vi "Stim Train Log String.vi"(1 "Single Channel Params":T1 {"Train Length" min=20 max=500 step=5}) -> (0 "Stim Train Log String":string)   [LabVIEW 2019]
uses:
  Controls/Type Defs/Single Channel Params.ctl
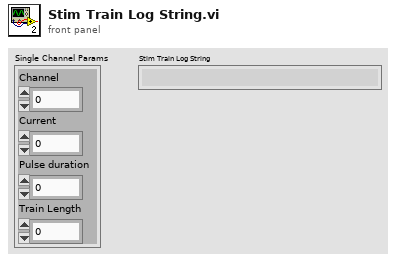
[diagram p1: front panel]
types:
  T1 = typedef "Single Channel Params.ctl" = cluster{"Channel":i32, "Current":u8, "Pulse duration":u16, "Train Length":i64}
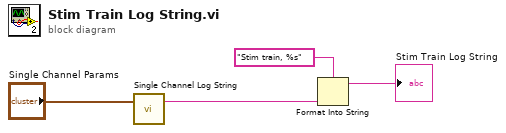
[diagram p0: block diagram]
diagram:
  n1 = call "Single Channel Log String.vi"("Single Channel Params"="Single Channel Params") -> ("Log String"=w2:string)  [unwired: 2 in]
  n2 = Format Into String(format string="Stim train, %s", w2) -> (resulting string=→"Stim Train Log String":string)  [unwired: 2 in, 1 out]
